vi "Configuration (Set).vi"   [LabVIEW 2013, in "Mercury iXX.lvlib"]
doc: "Set configuration data of the Mercury instrument or any devices within the system."
uses:
  <instrlib>/Mercury iXX/Mercury iXX.lvlib
  <instrlib>/Mercury iXX/Public/Libraries/System.lvlib
  <instrlib>/Mercury iXX/Public/Libraries/Temperature.lvlib
  <instrlib>/Mercury iXX/Public/Libraries/Heater.lvlib
  <instrlib>/Mercury iXX/Public/Libraries/Control Loop.lvlib
  <instrlib>/Mercury iXX/Public/Libraries/Level Meter.lvlib
  <instrlib>/Mercury iXX/Public/Libraries/Auxiliary.lvlib
  <instrlib>/Mercury iXX/Public/Libraries/Magnet.lvlib
  <instrlib>/Mercury iXX/Public/Libraries/Flow.lvlib
  <instrlib>/Mercury iXX/Public/Libraries/Pressure.lvlib
  <instrlib>/Mercury iXX/Public/Libraries/Lambda.lvlib
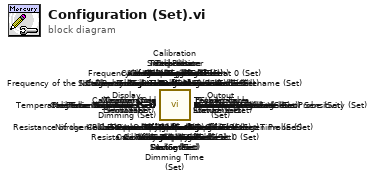
[diagram p0: block diagram]
diagram:
  n1 = call <instrlib>:"Lambda Percentage Flow (Set).vi"() -> ()  [unwired: 8 in, 4 out]
  n2 = call <instrlib>:"Lambda Flow Auto (Set).vi"() -> ()  [unwired: 8 in, 4 out]
  n3 = call <instrlib>:"Pulse Slow-Fast (Set).vi"() -> ()  [unwired: 8 in, 4 out]
  n4 = call <instrlib>:"Temperature Limit (Set).vi"() -> ()  [unwired: 8 in, 4 out]
  n5 = call <instrlib>:"Level Limit (Set).vi"() -> ()  [unwired: 8 in, 4 out]
  n6 = call <instrlib>:"Display Brightness (Set).vi"() -> ()  [unwired: 8 in, 4 out]
  n7 = call <instrlib>:"Display Automatic Dimming Time (Set).vi"() -> ()  [unwired: 8 in, 4 out]
  n8 = call <instrlib>:"Display Automatic Dimming (Set).vi"() -> ()  [unwired: 8 in, 4 out]
  n9 = call <instrlib>:"Calibrate (Set).vi"() -> ()  [unwired: 8 in, 4 out]
  n10 = call <instrlib>:"Nickname (Set).vi"() -> ()  [unwired: 8 in, 4 out]
  n11 = call <instrlib>:"Nickname (Set).vi"() -> ()  [unwired: 8 in, 4 out]
  n12 = call <instrlib>:"PSU Action Status (Set).vi"() -> ()  [unwired: 8 in, 4 out]
  n13 = call <instrlib>:"Pressure Sensor (Set).vi"() -> ()  [unwired: 8 in, 4 out]
  n14 = call <instrlib>:"Pressure Device (Set).vi"() -> ()  [unwired: 8 in, 4 out]
  n15 = call <instrlib>:"Nickname (Set).vi"() -> ()  [unwired: 8 in, 4 out]
  n16 = call <instrlib>:"Calibration Scaling (Set).vi"() -> ()  [unwired: 8 in, 4 out]
  n17 = call <instrlib>:"Calibration Offset (Set).vi"() -> ()  [unwired: 8 in, 4 out]
  n18 = call <instrlib>:"Calibration Low Limit (Set).vi"() -> ()  [unwired: 8 in, 4 out]
  n19 = call <instrlib>:"Calibration Interpolation (Set).vi"() -> ()  [unwired: 8 in, 4 out]
  n20 = call <instrlib>:"Calibration High Limit (Set).vi"() -> ()  [unwired: 8 in, 4 out]
  n21 = call <instrlib>:"Calibration Filename (Set).vi"() -> ()  [unwired: 8 in, 4 out]
  n22 = call <instrlib>:"Calibration Calibrate (Set).vi"() -> ()  [unwired: 8 in, 4 out]
  n23 = call <instrlib>:"Voltage Limit (Set).vi"() -> ()  [unwired: 8 in, 4 out]
  n24 = call <instrlib>:"Nominal Resistance (Set).vi"() -> ()  [unwired: 8 in, 4 out]
  n25 = call <instrlib>:"Nickname (Set).vi"() -> ()  [unwired: 8 in, 4 out]
  n26 = call <instrlib>:"Flow Device (Set).vi"() -> ()  [unwired: 8 in, 4 out]
  n27 = call <instrlib>:"Fastcool Mode (Set).vi"() -> ()  [unwired: 8 in, 4 out]
  n28 = call <instrlib>:"Calibrate (Set).vi"() -> ()  [unwired: 8 in, 4 out]
  n29 = call <instrlib>:"Flow Auto (Set).vi"() -> ()  [unwired: 8 in, 4 out]
  n30 = call <instrlib>:"Percentage Flow (Set).vi"() -> ()  [unwired: 8 in, 4 out]
  n31 = call <instrlib>:"Sweep Mode (Set).vi"() -> ()  [unwired: 8 in, 4 out]
  n32 = call <instrlib>:"Sweep Table Filename (Set).vi"() -> ()  [unwired: 8 in, 4 out]
  n33 = call <instrlib>:"Target Heater Table Filename (Set).vi"() -> ()  [unwired: 8 in, 4 out]
  n34 = call <instrlib>:"Auto PID Filename (Set).vi"() -> ()  [unwired: 8 in, 4 out]
  n35 = call <instrlib>:"Calibration Calibrate (Set).vi"() -> ()  [unwired: 8 in, 4 out]
  n36 = call <instrlib>:"Calibration Cold Limit (Set).vi"() -> ()  [unwired: 8 in, 4 out]
  n37 = call <instrlib>:"Calibration Hot Limit (Set).vi"() -> ()  [unwired: 8 in, 4 out]
  n38 = call <instrlib>:"Ignore Voltage Transient Time (Set).vi"() -> ()  [unwired: 8 in, 4 out]
  n39 = call <instrlib>:"Software Voltage Limit (Set).vi"() -> ()  [unwired: 8 in, 4 out]
  n40 = call <instrlib>:"Switch Heater Current (Set).vi"() -> ()  [unwired: 8 in, 4 out]
  n41 = call <instrlib>:"Switch Present (Set).vi"() -> ()  [unwired: 8 in, 4 out]
  n42 = call <instrlib>:"Magnetic Inductance (Set).vi"() -> ()  [unwired: 8 in, 4 out]
  n43 = call <instrlib>:"Current to Field Factor (Set).vi"() -> ()  [unwired: 8 in, 4 out]
  n44 = call <instrlib>:"Current Limit (Set).vi"() -> ()  [unwired: 8 in, 4 out]
  n45 = call <instrlib>:"Output Configuration (Set).vi"() -> ()  [unwired: 8 in, 4 out]
  n46 = call <instrlib>:"Bipolar Output (Set).vi"() -> ()  [unwired: 8 in, 4 out]
  n47 = call <instrlib>:"Nickname (Set).vi"() -> ()  [unwired: 8 in, 4 out]
  n48 = call <instrlib>:"Magnet Device (Set).vi"() -> ()  [unwired: 8 in, 4 out]
  n49 = call <instrlib>:"Stepper Speed (Set).vi"() -> ()  [unwired: 8 in, 4 out]
  n50 = call <instrlib>:"Valve Gearing (Set).vi"() -> ()  [unwired: 8 in, 4 out]
  n51 = call <instrlib>:"Temperature Voltage Error Sensitivity (Set).vi"() -> ()  [unwired: 8 in, 4 out]
  n52 = call <instrlib>:"Temperature Error Sensitivity (Set).vi"() -> ()  [unwired: 8 in, 4 out]
  n53 = call <instrlib>:"Gas Flow Scaling (Set).vi"() -> ()  [unwired: 8 in, 4 out]
  n54 = call <instrlib>:"Minimum Gas Flow (Set).vi"() -> ()  [unwired: 8 in, 4 out]
  n55 = call <instrlib>:"Aux Device (Set).vi"() -> ()  [unwired: 8 in, 4 out]
  n56 = call <instrlib>:"Level Meter Device (Set).vi"() -> ()  [unwired: 8 in, 4 out]
  n57 = call <instrlib>:"Nitrogen Pulse Count Period (Set).vi"() -> ()  [unwired: 8 in, 4 out]
  n58 = call <instrlib>:"Frequency of the Nitrogen Probe at 100 (Set).vi"() -> ()  [unwired: 8 in, 4 out]
  n59 = call <instrlib>:"Frequency of the Nitrogen Probe at 0 (Set).vi"() -> ()  [unwired: 8 in, 4 out]
  n60 = call <instrlib>:"Frequency of the Nitrogen Probe (Set).vi"() -> ()  [unwired: 8 in, 4 out]
  n61 = call <instrlib>:"Pulse Delay (Set).vi"() -> ()  [unwired: 8 in, 4 out]
  n62 = call <instrlib>:"Pulse Duration (Set).vi"() -> ()  [unwired: 8 in, 4 out]
  n63 = call <instrlib>:"Pulse Magnitude (Set).vi"() -> ()  [unwired: 8 in, 4 out]
  n64 = call <instrlib>:"Pre-Pulse Duration (Set).vi"() -> ()  [unwired: 8 in, 4 out]
  n65 = call <instrlib>:"Pre-Pulse Magnitude (Set).vi"() -> ()  [unwired: 8 in, 4 out]
  n66 = call <instrlib>:"Resistance of the Helium Probe at 100 (Set).vi"() -> ()  [unwired: 8 in, 4 out]
  n67 = call <instrlib>:"Resistance of the Helium Probe at 0 (Set).vi"() -> ()  [unwired: 8 in, 4 out]
  n68 = call <instrlib>:"Resistance of the Helium Probe (Set).vi"() -> ()  [unwired: 8 in, 4 out]
  n69 = call <instrlib>:"D Value (Set).vi"() -> ()  [unwired: 8 in, 4 out]
  n70 = call <instrlib>:"I Value (Set).vi"() -> ()  [unwired: 8 in, 4 out]
  n71 = call <instrlib>:"P Value (Set).vi"() -> ()  [unwired: 8 in, 4 out]
  n72 = call <instrlib>:"PID (Set).vi"() -> ()  [unwired: 8 in, 4 out]
  n73 = call <instrlib>:"PID Auto (Set).vi"() -> ()  [unwired: 8 in, 4 out]
  n74 = call <instrlib>:"Temperature Setpoint (Set).vi"() -> ()  [unwired: 8 in, 4 out]
  n75 = call <instrlib>:"Percentage Heat (Set).vi"() -> ()  [unwired: 8 in, 4 out]
  n76 = call <instrlib>:"Heater Auto (Set).vi"() -> ()  [unwired: 8 in, 4 out]
  n77 = call <instrlib>:"Level Association (Set).vi"() -> ()  [unwired: 8 in, 4 out]
  n78 = call <instrlib>:"Auxiliary Association (Set).vi"() -> ()  [unwired: 8 in, 4 out]
  n79 = call <instrlib>:"Heater Association (Set).vi"() -> ()  [unwired: 8 in, 4 out]
  n80 = call <instrlib>:"Control Loop (Set).vi"() -> ()  [unwired: 8 in, 4 out]
  n81 = call <instrlib>:"Mode (Set).vi"() -> ()  [unwired: 8 in, 4 out]
  n82 = call <instrlib>:"Heater Device (Set).vi"() -> ()  [unwired: 8 in, 4 out]
  n83 = call <instrlib>:"Temperature Device (Set).vi"() -> ()  [unwired: 8 in, 4 out]
  n84 = call <instrlib>:"Nominal Resistance (Set).vi"() -> ()  [unwired: 8 in, 4 out]
  n85 = call <instrlib>:"Voltage Limit (Set).vi"() -> ()  [unwired: 8 in, 4 out]
  n86 = call <instrlib>:"Nickname (Set).vi"() -> ()  [unwired: 8 in, 4 out]
  n87 = call <instrlib>:"Calibration Offset (Set).vi"() -> ()  [unwired: 8 in, 4 out]
  n88 = call <instrlib>:"Calibration Scaling (Set).vi"() -> ()  [unwired: 8 in, 4 out]
  n89 = call <instrlib>:"Calibration Interpolation (Set).vi"() -> ()  [unwired: 8 in, 4 out]
  n90 = call <instrlib>:"Calibration Filename (Set).vi"() -> ()  [unwired: 8 in, 4 out]
  n91 = call <instrlib>:"Excitation Magnitude (Set).vi"() -> ()  [unwired: 8 in, 4 out]
  n92 = call <instrlib>:"Excitation Type (Set).vi"() -> ()  [unwired: 8 in, 4 out]
  n93 = call <instrlib>:"Temperature Sensor (Set).vi"() -> ()  [unwired: 8 in, 4 out]
  n94 = call <instrlib>:"Nickname (Set).vi"() -> ()  [unwired: 8 in, 4 out]
  n95 = call <instrlib>:"Reset (Set).vi"() -> ()  [unwired: 8 in, 4 out]
  n96 = call <instrlib>:"DateTime (Set).vi"() -> ()  [unwired: 8 in, 4 out]
  n97 = call <instrlib>:"Time (Set).vi"() -> ()  [unwired: 8 in, 4 out]
  n98 = call <instrlib>:"Date (Set).vi"() -> ()  [unwired: 8 in, 4 out]
